vi "Loop Test.vi"(9 "Min":dbl=0.9, 10 "Max":dbl=1.2, 11 "Data Str":string="[ 1,1 1,2 1,3 1,4 1,6 ]") -> (3 "Result":bool)   [LabVIEW 2018]
uses:
  <vilib>/regexp/Match Regular Expression.xnode
panel:
  out "val 5":dbl
  out "val 4":dbl
  out "val 3":dbl
  out "val 2":dbl
  out "val 1":dbl
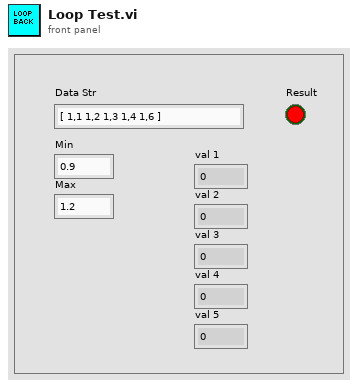
[diagram p1: front panel]
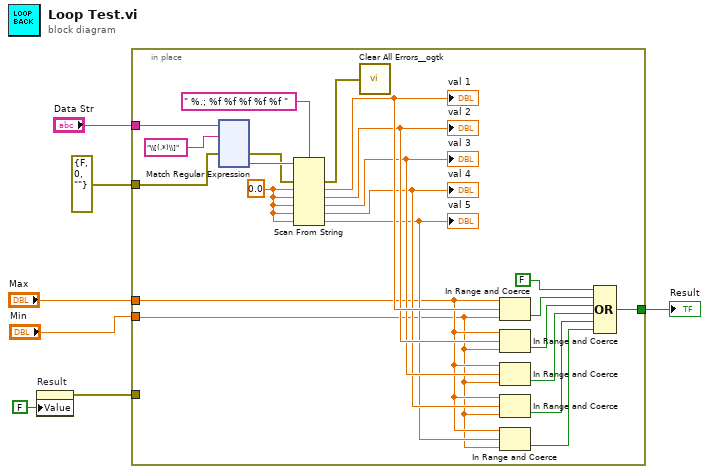
[diagram p0: block diagram]
diagram:
  n1 = property on="Result" class="Bool (strict)"("Value"=FALSE ("Result")) -> (error out=w6:errorcluster)  [unwired: 2 in, 1 out]
  n2 = in-place {
    in-place-border: w6 -> [_]
    in-place-border: "Data Str" -> [w29]
    in-place-border: errorcluster {"status"=FALSE, "code"=0, "source"=""} ("error in (no error)") -> [w25]
    in-place-border: "Max" -> [w17]
    in-place-border: "Min" -> [w16]
    in-place-border: [w9] -> w2
    w23 = 0.0
    n3 = xnode "Match Regular Expression"("input string"=w29, "regular expression"="\\[(.*)\\]", "error in"=w25) -> ("error out"=w24:errorcluster, "submatch 1"=w28:string)  [unwired: 3 in, 4 out]
    n4 = Scan From String(format string=" %.; %f %f %f %f %f ", input string=w28, error in=w24, default 1=w23, default 2=w23, default 3=w23, default 4=w23, default 5=w23) -> (error out=w8:errorcluster, output 1=w22:dbl, output 2=w21:dbl, output 3=w20:dbl, output 4=w19:dbl, output 5=w18:dbl)  [unwired: 1 in, 2 out]
    "val 1" <- w22
    "val 2" <- w21
    "val 3" <- w20
    "val 4" <- w19
    "val 5" <- w18
    n5 = call <userlib>:"Clear All Errors__ogtk.vi"("Error In"=w8) -> ()  [unwired: 3 in, 1 out]
    n6 = In Range and Coerce(upper limit=w17, x=w22, lower limit=w16) -> (In Range?=w14:bool)  [unwired: 1 out]
    n7 = In Range and Coerce(upper limit=w17, x=w21, lower limit=w16) -> (In Range?=w13:bool)  [unwired: 1 out]
    n8 = In Range and Coerce(upper limit=w17, x=w20, lower limit=w16) -> (In Range?=w12:bool)  [unwired: 1 out]
    n9 = In Range and Coerce(upper limit=w17, x=w19, lower limit=w16) -> (In Range?=w11:bool)  [unwired: 1 out]
    n10 = In Range and Coerce(upper limit=w17, x=w18, lower limit=w16) -> (In Range?=w10:bool)  [unwired: 1 out]
    n11 = Compound Arithmetic op=OR(FALSE, w14, w13, w12, w11, w10) -> (w9:bool)
  }
  "Result" <- w2
